vi "Joystick Values.vi"(1 "Joystick Index":i32=2 min=2 max=5 step=1) -> (0 "Joystick":T1)   [LabVIEW 2014]
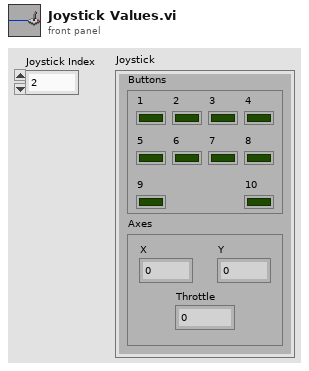
[diagram p1: front panel]
types:
  T1 = cluster{"Buttons":cluster{"1":bool, "2":bool, "3":bool, "4":bool, "5":bool, "6":bool, "7":bool, "8":bool, "9":bool, "10":bool}, "Axes":cluster{"X":dbl, "Y":dbl, "Throttle":dbl}}
  T2 = cluster{"Boolean":bool, "Boolean":bool, "Boolean":bool, "Boolean":bool, "Boolean":bool, "Boolean":bool, "Boolean":bool, "Boolean":bool, "Boolean":bool, "Boolean":bool}
  T3 = cluster{"Numeric":dbl, "Numeric":dbl, "Numeric":dbl}
  T4 = cluster{cluster{"Boolean":bool, "Boolean":bool, "Boolean":bool, "Boolean":bool, "Boolean":bool, "Boolean":bool, "Boolean":bool, "Boolean":bool, "Boolean":bool, "Boolean":bool}, cluster{"Numeric":dbl, "Numeric":dbl, "Numeric":dbl}}
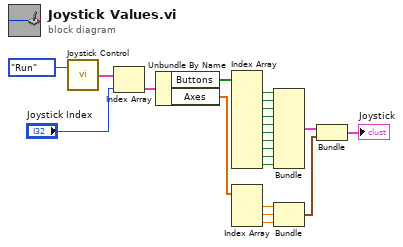
[diagram p0: block diagram]
diagram:
  n1 = call "Joystick Control.vi"("Mode"=enum8{"Start", "Run", "Finish"}."Run") -> ("Joysticks"=w21:cluster{"Buttons":bool[], "Axes":dbl[]}[])  [unwired: 1 in]
  n2 = Index Array(array=w21, index="Joystick Index") -> (element=w20:cluster{"Buttons":bool[], "Axes":dbl[]})
  n3 = Unbundle By Name(w20) -> ("Buttons"=w19:bool[], "Axes"=w8:dbl[])
  n4 = Index Array(array=w19) -> (element #1=w17:bool, element #2=w18:bool, element #3=w9:bool, element #4=w10:bool, element #5=w11:bool, element #6=w12:bool, element #7=w13:bool, element #8=w14:bool, element #9=w15:bool, element #10=w16:bool)  [unwired: 10 in]
  n5 = Index Array(array=w8) -> (element #1=w6:dbl, element #2=w7:dbl, element #3=w5:dbl)  [unwired: 3 in]
  n6 = Bundle("Boolean"=w17, "Boolean"=w18, "Boolean"=w9, "Boolean"=w10, "Boolean"=w11, "Boolean"=w12, "Boolean"=w13, "Boolean"=w14, "Boolean"=w15, "Boolean"=w16) -> (w4:T2)  [unwired: 1 in]
  n7 = Bundle("Numeric"=w6, "Numeric"=w7, "Numeric"=w5) -> (w3:T3)  [unwired: 1 in]
  n8 = Bundle(w4, w3) -> (→"Joystick":T4)  [unwired: 1 in]
